vi "_AnalyzeErrors.vi"() -> ()   [LabVIEW 2012]
panel:
  in  "stop":bool
  out "Total Server Errors":i32
  out "Total Console Errors":i32
  in  "Tab Control":enum32{"Console Errors", "Server Errors"}(tab)
  out "Console Errors":T1(array[cluster])
  out "Cmd Log":T2(array[cluster])
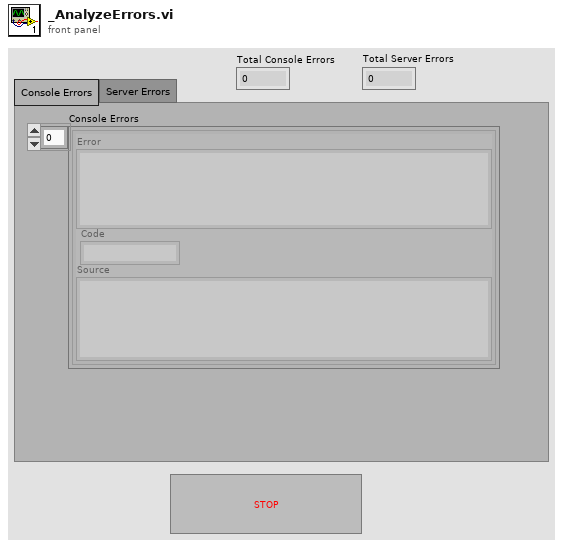
[diagram p1: front panel]
types:
  T1 = cluster{"Error":string, "Code":string, "Source":string}[]
  T2 = cluster{"Sent":string, "Reply":string, "MethodName":string, "success":bool, "Dir1":string, "Dir2":string, "Time Stamp":string, "Error":string, "VI":string}[]
  T3 = cluster{"Sent":string, "Reply":string, "MethodName":string, "success":bool, "Dir1":string, "Dir2":string, "Time Stamp":string, "Error":string, "VI":string}
  T4 = cluster{"Error":string, "Code":string, "Source":string}
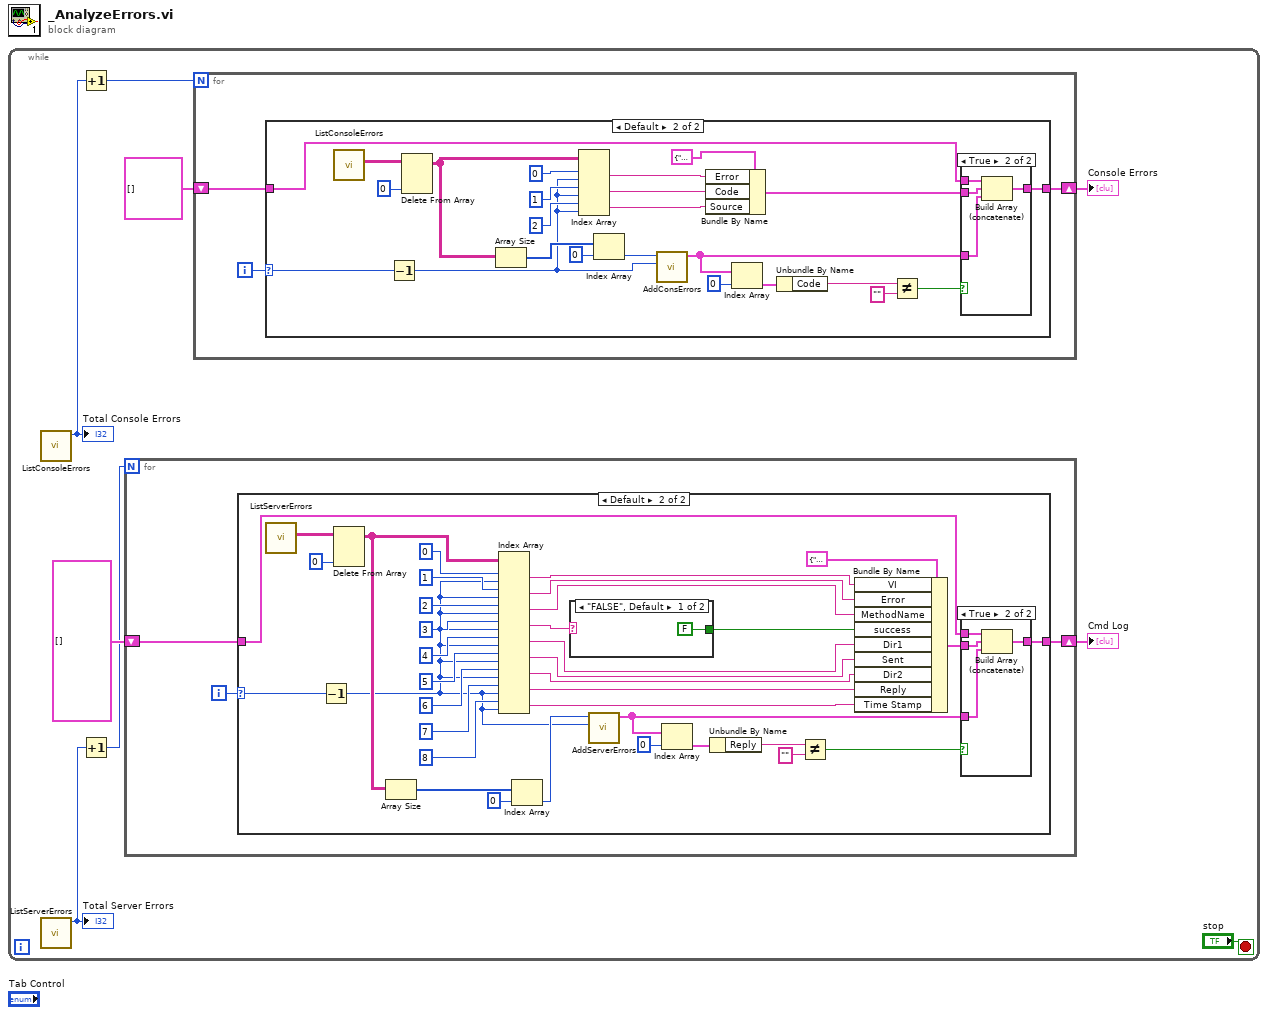
[diagram p0: block diagram]
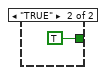
[diagram p3: hidden frame]
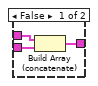
[diagram p4: hidden frame]
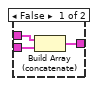
[diagram p6: hidden frame]
diagram:
  n1 = while {
    stop <- "stop" stop-if-true
    n2 = call <userlib>:"ListConsoleErrors.vi"() -> ("Total Console Errors"=w1:i32)  [unwired: 10 in, 1 out]
    "Total Console Errors" <- w1
    n3 = call <userlib>:"ListServerErrors.vi"() -> ("Total Server Errors"=w3:i32)  [unwired: 10 in, 1 out]
    "Total Server Errors" <- w3
    n4 = Increment(x=w1) -> (x+1=w2:i32)
    n5 = Increment(x=w3) -> (x+1=w4:i32)
    n6 = for {
      N: w4 -> [_]
      shift-right: [w10] -> w5
      shift-left: T2 [] ("Cmd Log") -> [w11]
      i -> [w12]
      n7 = case shown="Default" w12 {
        selector: w12 -> [_ w37]
        tunnel: w11 -> [w13 w44]
        tunnel: [w13 w42] -> w10
        frame 0 {
        }
        frame Default {
          n8 = call <userlib>:"ListServerErrors.vi"() -> ("Array"=w30:string[][])  [unwired: 10 in, 1 out]
          n9 = Decrement(x=w37) -> (x-1=w15:i32)
          n10 = Delete From Array(array=w30, index (col)=0 ("disabled index (col)")) -> (array with subset deleted=w38:string[][])  [unwired: 2 in, 1 out]
          n11 = Array Size(array=w38) -> (size(s)=w47:i32[])
          n12 = Index Array(array=w38, index (row) #1=0 ("index (row)"), index (col) #1=w15, index (row) #2=1 ("index (row)"), index (col) #2=w15, index (row) #3=2 ("index (row)"), index (col) #3=w15, index (row) #4=3 ("index (row)"), index (col) #4=w15, index (row) #5=4 ("index (row)"), index (col) #5=w15, index (row) #6=5 ("index (row)"), index (col) #6=w15, index (row) #7=6 ("index (row)"), index (col) #7=w15, index (row) #8=7 ("index (row)"), index (col) #8=w15, index (row) #9=8 ("index (row)"), index (col) #9=w15) -> (element #1=w14:string, element #2=w40:string, element #3=w41:string, element #4=w29:string, element #5=w22:string, element #6=w21:string, element #7=w20:string, element #8=w19:string, element #9=w18:string)
          n13 = Index Array(array=w47, index=0) -> (element=w45:i32)
          n14 = case shown="\"FALSE\", Default" w29 {
            tunnel: [FALSE TRUE] -> w28
            frame "FALSE", Default {
            }
            frame "TRUE" {
            }
          }
          n15 = call <userlib>:"AddServerErrors.vi"("Numeric"=w15, "Numeric 2"=w45) -> ("Cmd Log"=w36:T2)  [unwired: 9 in]
          n16 = Index Array(array=w36, index=0) -> (element=w33:T3)
          n17 = Unbundle By Name(w33) -> ("Reply"=w32:string)
          n18 = Not Equal?(x=w32, y="") -> (x != y?=w34:bool)
          n19 = Bundle By Name(cluster=T3 {"Sent"="", "Reply"="", "MethodName"="", "success"=FALSE, "Dir1"="", "Dir2"="", "Time Stamp"="", "Error"="", "VI"=""} ("Log"), "VI"=w14, "Error"=w40, "MethodName"=w41, "success"=w28, "Dir1"=w22, "Sent"=w21, "Dir2"=w20, "Reply"=w19, "Time Stamp"=w18) -> (w43:T3)
          n20 = case shown="True" w34 {
            tunnel: w44 -> [w54 w59]
            tunnel: w43 -> [w55 w58]
            tunnel: [w53 w57] -> w42
            tunnel: w36 -> [_ w56]
            frame False {
              n21 = Build Array (concatenate)(w54, w55) -> (w53:T2)
            }
            frame True {
              n22 = Build Array (concatenate)(w59, w58, w56) -> (w57:T2)
            }
          }
        }
      }
    }
    "Cmd Log" <- w5
    n23 = for {
      N: w2 -> [_]
      shift-right: [w60] -> w7
      shift-left: T1 [] ("Array 2") -> [w61]
      i -> [w62]
      n24 = case shown="Default" w62 {
        selector: w62 -> [_ w72]
        tunnel: w61 -> [w63 w81]
        tunnel: [w63 w79] -> w60
        frame 0 {
        }
        frame Default {
          n25 = call <userlib>:"ListConsoleErrors.vi"() -> ("Array"=w75:string[][])  [unwired: 10 in, 1 out]
          n26 = Decrement(x=w72) -> (x-1=w65:i32)
          n27 = Delete From Array(array=w75, index (col)=0 ("disabled index (col)")) -> (array with subset deleted=w73:string[][])  [unwired: 2 in, 1 out]
          n28 = Array Size(array=w73) -> (size(s)=w83:i32[])
          n29 = Index Array(array=w73, index (row) #1=0 ("index (row)"), index (col) #1=w65, index (row) #2=1 ("index (row)"), index (col) #2=w65, index (row) #3=2 ("index (row)"), index (col) #3=w65) -> (element #1=w77:string, element #2=w78:string, element #3=w76:string)
          n30 = Index Array(array=w83, index=0) -> (element=w66:i32)
          n31 = call <userlib>:"AddConsErrors.vi"("Numeric"=w65, "Numeric 2"=w66) -> ("Array 2"=w64:T1)  [unwired: 9 in]
          n32 = Bundle By Name(cluster=T4 {"Error"="", "Code"="", "Source"=""} ("ConsoleError"), "Error"=w77, "Code"=w78, "Source"=w76) -> (w80:T4)
          n33 = Index Array(array=w64, index=0) -> (element=w69:T4)
          n34 = Unbundle By Name(w69) -> ("Code"=w68:string)
          n35 = Not Equal?(x=w68, y="") -> (x != y?=w70:bool)
          n36 = case shown="True" w70 {
            tunnel: w81 -> [w89 w94]
            tunnel: w80 -> [w90 w93]
            tunnel: [w88 w92] -> w79
            tunnel: w64 -> [_ w91]
            frame False {
              n37 = Build Array (concatenate)(w89, w90) -> (w88:T1)
            }
            frame True {
              n38 = Build Array (concatenate)(w94, w93, w91) -> (w92:T1)
            }
          }
        }
      }
    }
    "Console Errors" <- w7
  }
